vi "客厅的面积.vi"() -> ()   [LabVIEW 2020]
panel:
  out "12.5ft变m并且不带单位":dbl=22.5
  out "22.5ft变m并且不带单位":dbl=22.5
  out "m^2":dbl[unit]
  out "12.5ft变m并且带单位":dbl[unit]
  out "22.5ft变m并且带单位":dbl[unit]
  out "m^2":dbl[unit]
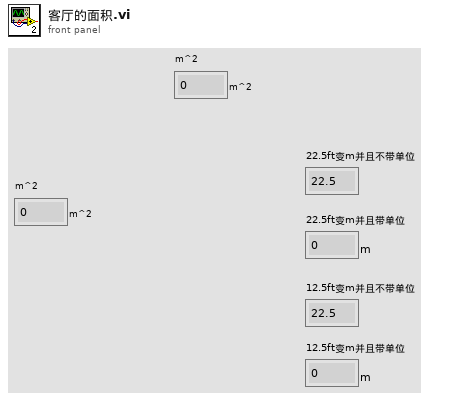
[diagram p1: front panel]
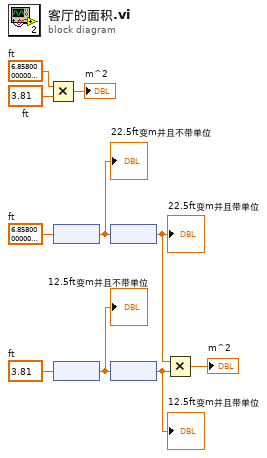
[diagram p0: block diagram]
diagram:
  w6 = dbl[unit] 3.81  # ft
  w7 = dbl[unit] 6.8580000000000005  # ft
  w9 = dbl[unit] 3.81  # ft
  w10 = dbl[unit] 6.8580000000000005  # ft
  n1 = Multiply(x=w10, y=w9) -> (x*y=→"m^2":dbl[unit])
  n2 = node(w7) -> (w2:dbl)
  "22.5ft变m并且不带单位" <- w2
  n3 = node(w6) -> (w1:dbl)
  "12.5ft变m并且不带单位" <- w1
  n4 = node(w2) -> (w4:dbl[unit])
  "22.5ft变m并且带单位" <- w4
  n5 = node(w1) -> (w3:dbl[unit])
  "12.5ft变m并且带单位" <- w3
  n6 = Multiply(x=w4, y=w3) -> (x*y=→"m^2":dbl[unit])
